vi "LEDs.vi"(10 "Reference":u32, 11 "Working":u32) -> (3 "Cluster":T1)   [LabVIEW 2015]
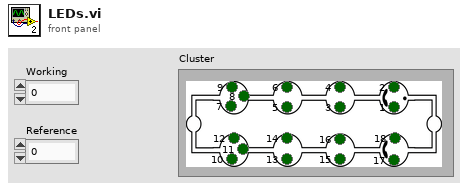
[diagram p1: front panel]
types:
  T1 = cluster{"1":bool, "2":bool, "3":bool, "4":bool, "5":bool, "6":bool, "7":bool, "8":bool, "9":bool, "10":bool, " 11":bool, " 12":bool, "13":bool, "14":bool, "15":bool, "16":bool, "17":bool, "18":bool}
  T2 = cluster{"[0]":bool, "[1]":bool, "[2]":bool, "[3]":bool, "[4]":bool, "[5]":bool, "[6]":bool, "[7]":bool, "[8]":bool, "[9]":bool, "[10]":bool, "[11]":bool, "[12]":bool, "[13]":bool, "[14]":bool, "[15]":bool, "[16]":bool, "[17]":bool, "[18]":bool}
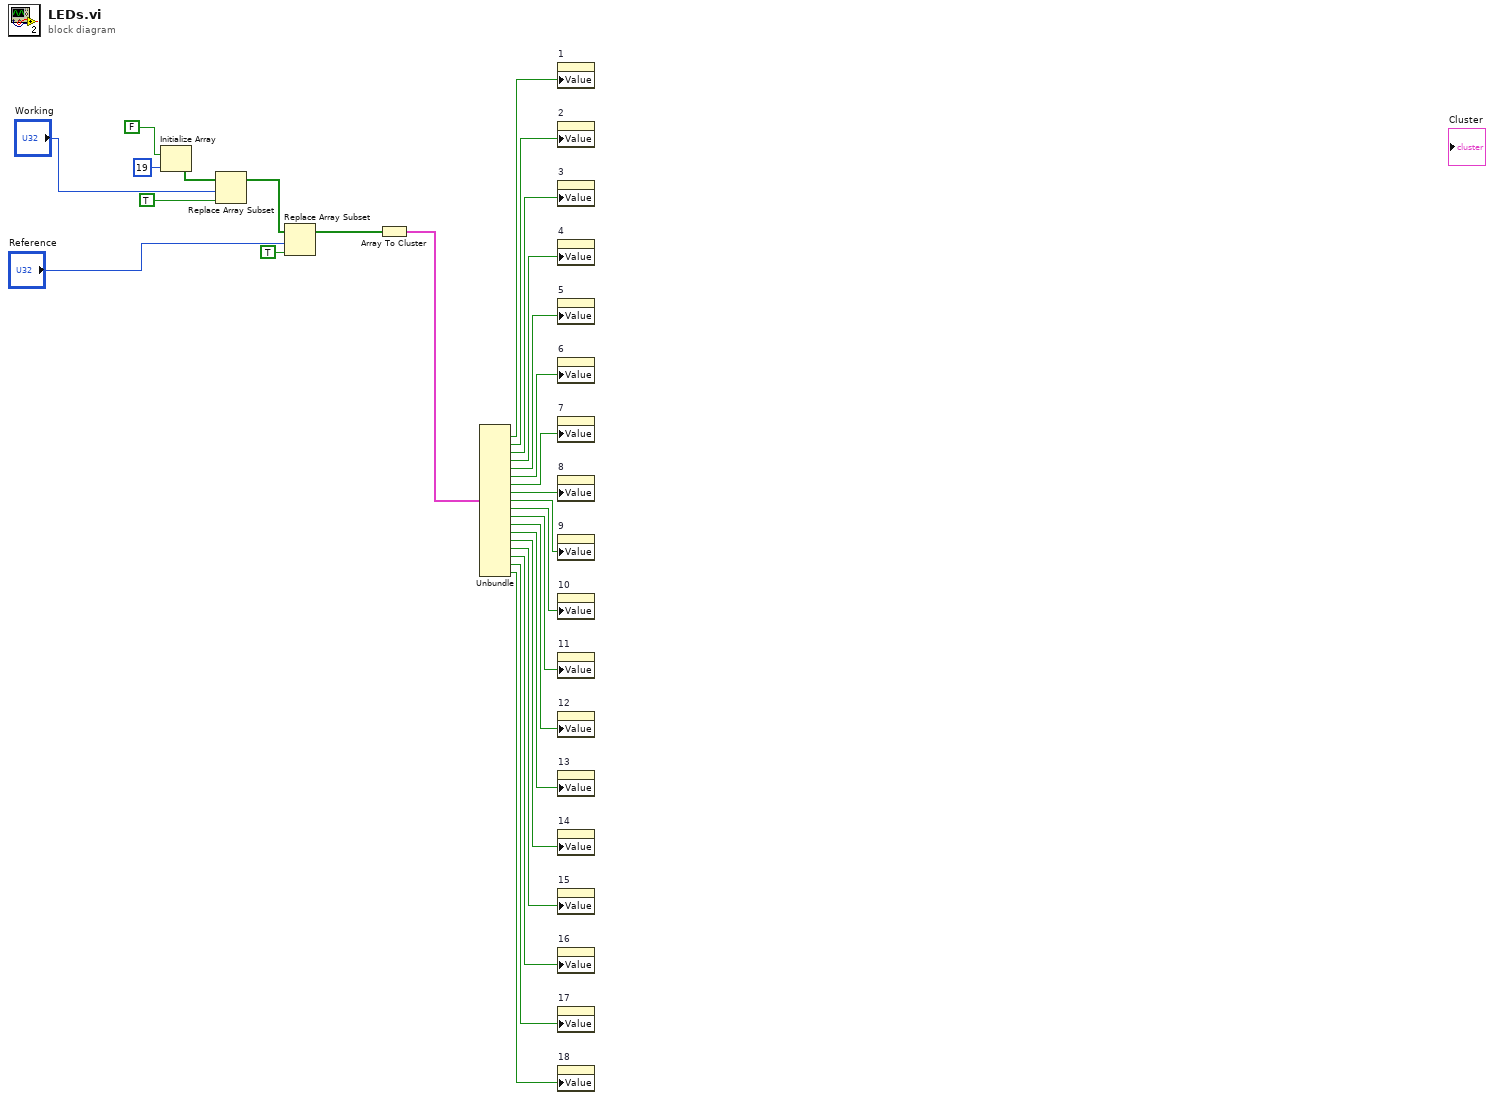
[diagram p0: block diagram]
diagram:
  n1 = Initialize Array(FALSE, 19 ("dimension size")) -> (w7:bool[])
  n2 = Replace Array Subset(array=w7, new element=TRUE ("new element/subarray"), index="Working") -> (w4:bool[])
  n3 = Replace Array Subset(array=w4, new element=TRUE ("new element/subarray"), index="Reference") -> (w2:bool[])
  n4 = Array To Cluster(array=w2) -> (cluster=w26:T2)
  n5 = Unbundle(w26) -> ("[1]"=w25:bool, "[2]"=w24:bool, "[3]"=w23:bool, "[4]"=w22:bool, "[5]"=w21:bool, "[6]"=w20:bool, "[7]"=w19:bool, "[8]"=w18:bool, "[9]"=w17:bool, "[10]"=w16:bool, "[11]"=w15:bool, "[12]"=w14:bool, "[13]"=w13:bool, "[14]"=w12:bool, "[15]"=w11:bool, "[16]"=w10:bool, "[17]"=w9:bool, "[18]"=w8:bool)  [unwired: 1 out]
  n6 = property on="1" class="Bool (strict)"("Value"=w25) -> ()  [unwired: 2 in, 2 out]
  n7 = property on="2" class="Bool (strict)"("Value"=w24) -> ()  [unwired: 2 in, 2 out]
  n8 = property on="3" class="Bool (strict)"("Value"=w23) -> ()  [unwired: 2 in, 2 out]
  n9 = property on="4" class="Bool (strict)"("Value"=w22) -> ()  [unwired: 2 in, 2 out]
  n10 = property on="5" class="Bool (strict)"("Value"=w21) -> ()  [unwired: 2 in, 2 out]
  n11 = property on="6" class="Bool (strict)"("Value"=w20) -> ()  [unwired: 2 in, 2 out]
  n12 = property on="7" class="Bool (strict)"("Value"=w19) -> ()  [unwired: 2 in, 2 out]
  n13 = property on="8" class="Bool (strict)"("Value"=w18) -> ()  [unwired: 2 in, 2 out]
  n14 = property on="9" class="Bool (strict)"("Value"=w17) -> ()  [unwired: 2 in, 2 out]
  n15 = property on="10" class="Bool (strict)"("Value"=w16) -> ()  [unwired: 2 in, 2 out]
  n16 = property on="11" class="Bool (strict)"("Value"=w15) -> ()  [unwired: 2 in, 2 out]
  n17 = property on="12" class="Bool (strict)"("Value"=w14) -> ()  [unwired: 2 in, 2 out]
  n18 = property on="13" class="Bool (strict)"("Value"=w13) -> ()  [unwired: 2 in, 2 out]
  n19 = property on="14" class="Bool (strict)"("Value"=w12) -> ()  [unwired: 2 in, 2 out]
  n20 = property on="15" class="Bool (strict)"("Value"=w11) -> ()  [unwired: 2 in, 2 out]
  n21 = property on="16" class="Bool (strict)"("Value"=w10) -> ()  [unwired: 2 in, 2 out]
  n22 = property on="17" class="Bool (strict)"("Value"=w9) -> ()  [unwired: 2 in, 2 out]
  n23 = property on="18" class="Bool (strict)"("Value"=w8) -> ()  [unwired: 2 in, 2 out]
